vi "graphOnScreen.vi"(6 "Connect to loop iteration":i32, 8 "Time":dbl, 9 "332 Temp [K]":dbl, 10 "332 Temp Setpoint [K]":dbl, 11 "R(ohm)":dbl) -> (0 "T(t)":cluster{"X":dbl, "Y":dbl}[](graph), 3 "?":cluster{dbl, dbl}[](graph))   [LabVIEW 2012]
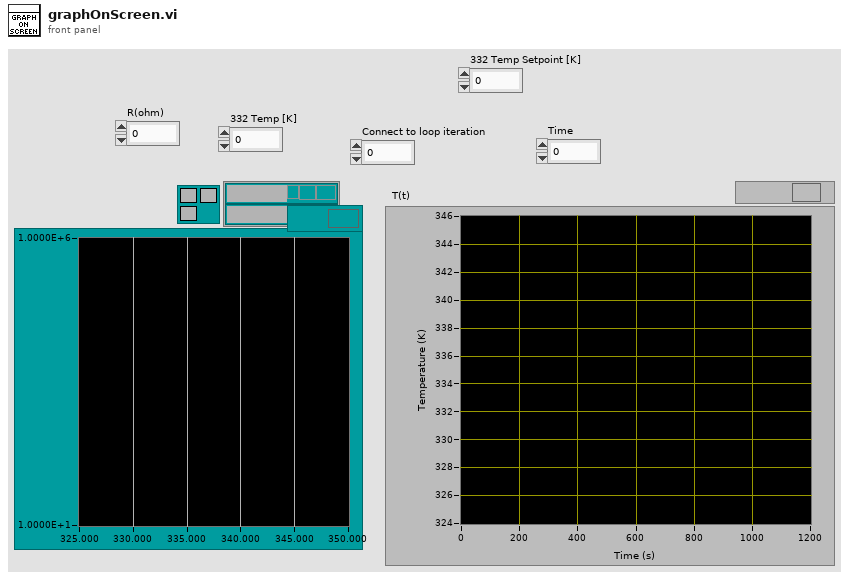
[diagram p1: front panel]
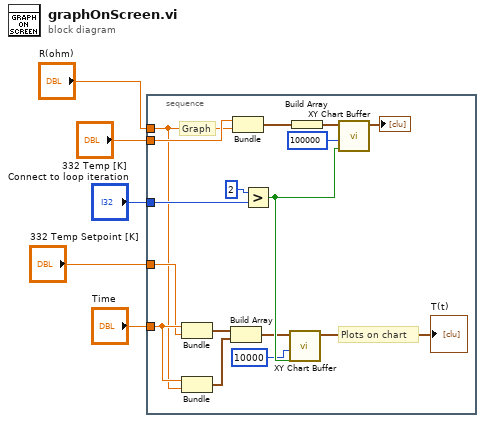
[diagram p0: block diagram]
diagram:
  n1 = stacked-sequence {
    tunnel: "Connect to loop iteration" -> [w17]
    tunnel: "R(ohm)" -> [w6]
    tunnel: "332 Temp [K]" -> [w15]
    tunnel: "Time" -> [w14]
    tunnel: "332 Temp Setpoint [K]" -> [w13]
    frame #0 {
      # "Plots on chart"
      # "Graph"
      n2 = Bundle("Time"=w14, "332 Temp Setpoint [K]"=w13) -> (w12:cluster{"Time":dbl, "332 Temp Setpoint [K]":dbl})  [unwired: 1 in]
      n3 = Bundle("Time"=w14, "R(ohm)"=w6) -> (w7:cluster{"Time":dbl, "R(ohm)":dbl})  [unwired: 1 in]
      n4 = Build Array(w12, w7) -> (w9:cluster{"Time":dbl, "R(ohm)":dbl}[])
      n5 = Bundle("332 Temp [K]"=w15, "R(ohm)"=w6) -> (w21:cluster{"332 Temp [K]":dbl, "R(ohm)":dbl})  [unwired: 1 in]
      n6 = Greater?(x=2, y=w17) -> (0:w11:bool)
      n7 = call "XY Chart Buffer.vi"("clear first (no:F)"=w11, "chart length (points)"=10000, "new points"=w9) -> ("XY chart data"=→"T(t)":cluster{"x":dbl, "y":dbl}[])  [unwired: 8 in]
      n8 = Build Array(w21) -> (w19:cluster{"332 Temp [K]":dbl, "R(ohm)":dbl}[])
      n9 = call "XY Chart Buffer.vi"("clear first (no:F)"=w11, "chart length (points)"=100000, "new points"=w19) -> ("XY chart data"=→"?":cluster{"x":dbl, "y":dbl}[])  [unwired: 8 in]
    }
  }
